vi "play_sysID_Z_Axis.vi"() -> ()   [LabVIEW 2017]
uses:
  sysID_Z-axis-params.ctl
  <vilib>/FPGAPlugInAG/cRIO-9082/niLvFpga_Open_cRIO-9082.vi
  <vilib>/rvi/interface/common/dynamic/niFpgaDynamicAddResources.vi
  <vilib>/FPGAPlugInAG/Dynamic/niLvFpga_Reset_Dynamic.vi
  <vilib>/rvi/interface/common/niFpgaWaitOnOcc.vi
  <vilib>/Utility/error.llb/Error Cluster From Error Code.vi
  <vilib>/rvi/errors/niLvFpgaAdjustHostInterfaceError.vi
  <vilib>/FPGAPlugInAG/Dynamic/niLvFpga_Run_Dynamic.vi
  <vilib>/FPGAPlugInAG/Dynamic/niLvFpga_Close_Dynamic.vi
  <vilib>/rvi/interface/nirviOpenFPGA/nirviOpenFPGA.xnode
  FPGA Bitfiles/afmimagingcontro_FPGATargetSPARTA_fpgasysIDZaxissi_jhd3Wt3fyx0.lvbitx
  <vilib>/rvi/interface/nirviMethod/nirviMethod.xnode
  <vilib>/rvi/interface/nirviReadWriteControl/nirviReadWriteControl.xnode
  <vilib>/rvi/interface/nirviCloseFPGA/nirviCloseFPGA.xnode
  <vilib>/FPGAPlugInAG/Dynamic/niLvFpga_ConfigureFifo_Dynamic.vi
  <vilib>/rvi/errors/niLvFpgaMergeErrorWithErrorCode.vi
  NiFpgaLv.dll
  <vilib>/rvi/interface/Simulation/niFpgaSimulationCallBeginRW.vi
panel:
  in  "Tab Control":enum32{"Main Control", "Debug Info"}(tab)
  in  "z-axis-settings":T1={"TOL"=0.3, "ramp-rate"=-5e-05, "z-u-max"=5.0, "offset"=0.0, "Ki"=0.001, "Z-error-threshold"=0.2, "Z-settled-samples\nthreshold "=200, "z_UP"=1.5, "zup-N"=5000} {"Z-error-threshold" format="%#_13g"; "ramp-rate" format="%#_4g"; "TOL" format="%#_13g"}
  in  "Z up":fxp<+/-,16,5>
  in  "trigger-0":bool
  in  "ABORT":bool
  out "Current Freq":dbl format="%#_13g"
  in  "Input Folder":path=path "C:/Users/arnold/Documents/MATLAB/AFM_SS/System_Identification/data/data_ZAxis"
  out "dataIn Path":path
  out "num_freqs":i32
  in  "input-file-name":string="z-axis_sines_in_299.csv"
  out "Input-meta-data-path":path
  out "output-data-path":path
  in  "overwrite":bool
  in  "note-blob":string
  out "Elements Remaining":i32=1
  out "Nsamps_i":i32
  out "size(s)":i32
  out "Current Case":i16
  out "log fifo num":i16
  out "input fifo num":i16
  out "error":errorcluster
  out "boolean  indicators 2":T2
  out "uzk)":dbl[](graph)
  out "z-err(k)":dbl[](graph)
  out "freqs":dbl[](array[numeric])
  out "ref(k) Signal":dbl[](graph)
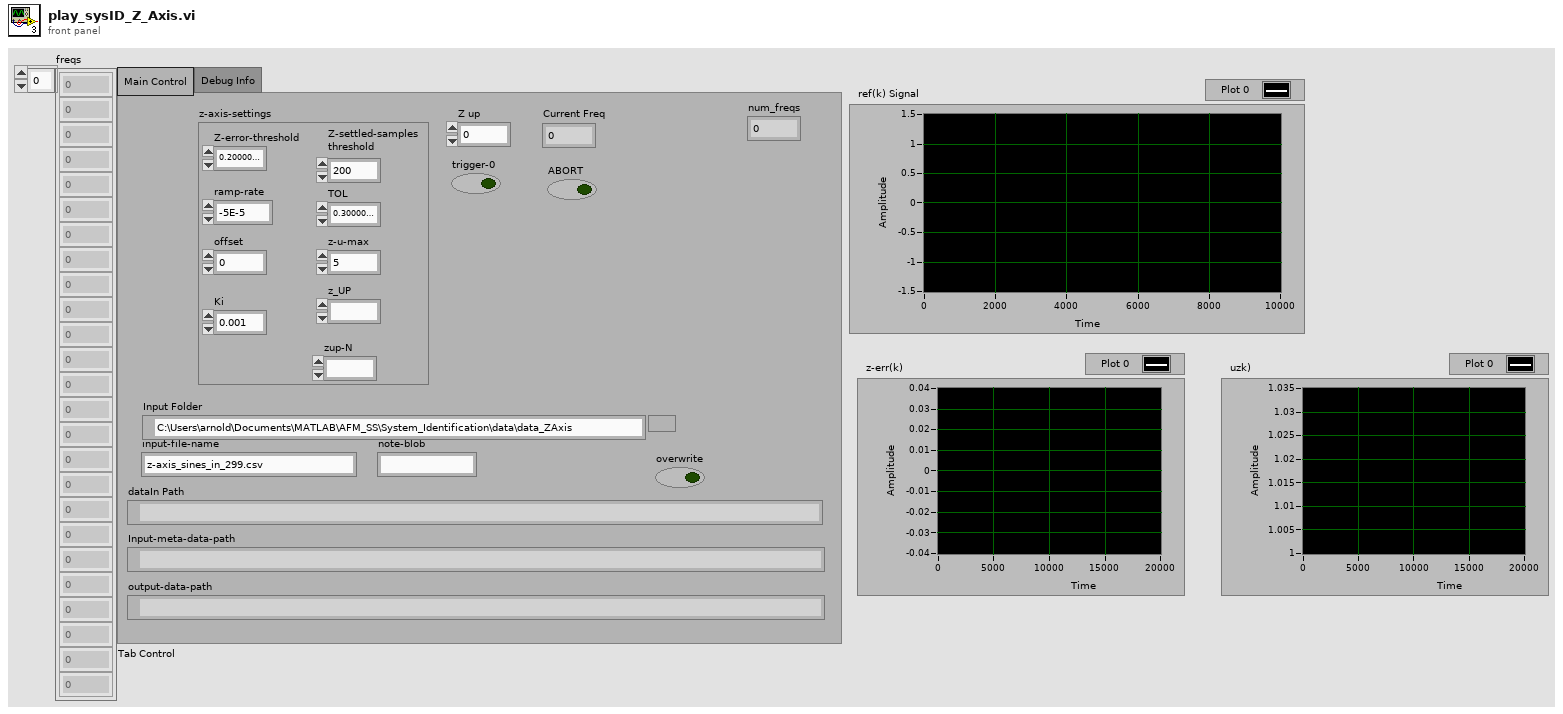
[diagram p1: front panel]
types:
  T1 = typedef "sysID_Z-axis-params.ctl" = cluster{"TOL":sgl, "ramp-rate":sgl, "z-u-max":sgl, "offset":sgl, "Ki":sgl, "Z-error-threshold":sgl, "Z-settled-samples\nthreshold ":i16, "z_UP":fxp<+/-,16,5>, "zup-N":i16}
  T2 = cluster{"unstable-z-traj":bool, "input fifo time-out":bool, "logging fifo timeout":bool, "scanning finished":bool, "unstable-x-traj":bool, "unstable-y-traj":bool, "ABORT":bool, "All Measurements Done":bool}
  T3 = typedef "sysID_ControlParams.ctl" = cluster{"Kp":sgl, "Umax ":sgl, "ymax":sgl, "TsTicks":u32, "z1":sgl, "num":sgl[], "den":sgl[], "TF Order":u8}
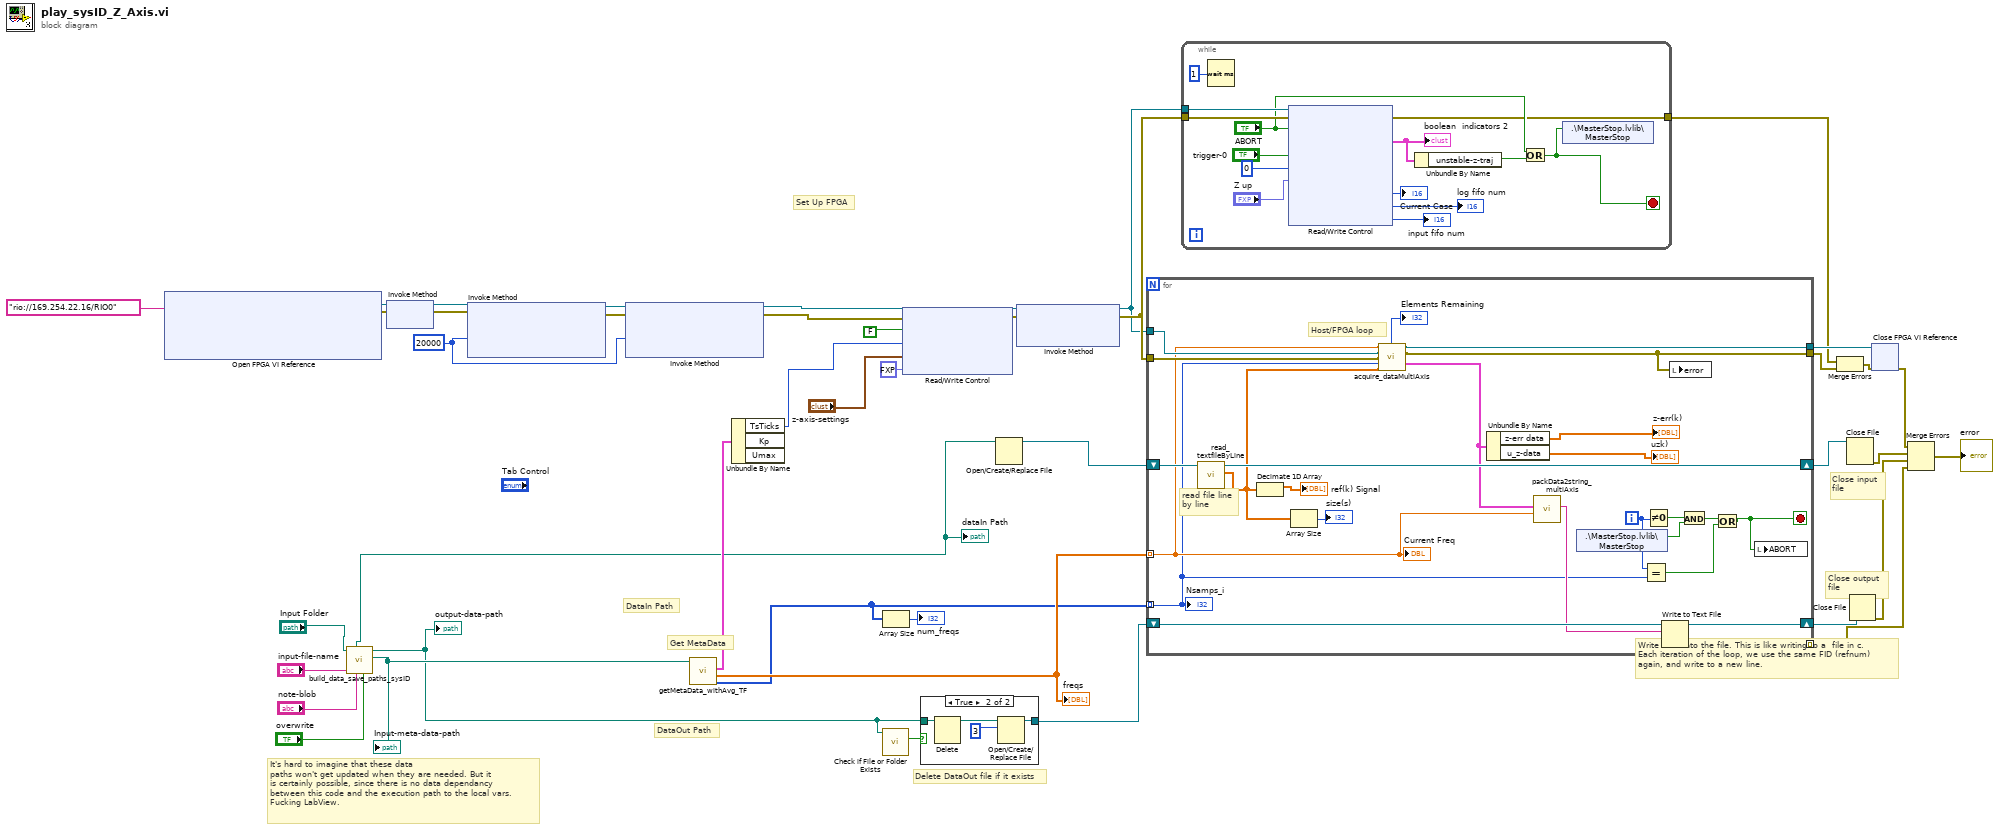
[diagram p0: block diagram]
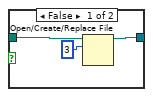
[diagram p2: hidden frame]
diagram:
  w14 = 20000 ("requested depth")
  # "It's hard to imagine that these data\npaths won't get updated when they are needed. But it \nis certainly possible, since there is no data dependancy \nbetween this code and the execution path to the local vars.\nFucking LabView."
  # "Set Up FPGA"
  # "Delete DataOut file if it exists"
  # "Close output\nfile"
  # "Close input\nfile"
  # "Write data into the file. This is like writing to a  file in c.\nEach iteration of the loop, we use the same FID (refnum) \nagain, and write to a new line."
  # "DataIn Path"
  # "DataOut Path"
  # "Get MetaData"
  n1 = xnode "Open FPGA VI Reference"("resource name"=tag "rio://169.254.22.16/RIO0") -> ("FPGA VI Reference Out"=w23:refnum<k20>, "error out"=w22:errorcluster)  [unwired: 1 in]
  n2 = call "build_data_save_paths_sysID.vi"("overwrite"="overwrite", "note-blob"="note-blob", "base-file-name"="input-file-name", "data-root"="Input Folder") -> ("output-meta-data-path"=w2:path, "output-data-path"=w1:path, "input-data-path"=w3:path)  [unwired: 4 in, 1 out]
  "dataIn Path" <- w3
  "Input-meta-data-path" <- w2
  "output-data-path" <- w1
  n3 = xnode "Invoke Method"("FPGA VI Reference In"=w23, "error in"=w22) -> ("FPGA VI Reference Out"=w27:refnum<k20>, "error out"=w26:errorcluster)
  n4 = xnode "Invoke Method"("FPGA VI Reference In"=w27, "error in"=w26, "Requested Depth"=w14) -> ("FPGA VI Reference Out"=w25:refnum<k20>, "error out"=w24:errorcluster)  [unwired: 1 out]
  n5 = xnode "Invoke Method"("FPGA VI Reference In"=w25, "error in"=w24, "Requested Depth"=w14) -> ("FPGA VI Reference Out"=w21:refnum<k20>, "error out"=w20:errorcluster)  [unwired: 1 out]
  n6 = call "getMetaData_withAvg_TF.vi"("MetaDataPath"=w2) -> ("Num Samples"=w9:i32[], "freqs (hz)"=w31:dbl[], "ControlParams"=w19:T3)  [unwired: 7 in]
  "freqs" <- w31
  n7 = Unbundle By Name(w19) -> ("TsTicks"=w15:u32)  [unwired: 2 out]
  n8 = call <vilib>:"Check if File or Folder Exists.vi"("path"=w1) -> ("file or folder exists?"=w28:bool)  [unwired: 8 in, 2 out]
  n9 = Array Size(array=w9) -> (size(s)=→"num_freqs":i32)
  n10 = xnode "Read/Write Control"("FPGA VI Reference In"=w21, "error in"=w20, "ABORT"=FALSE, "TsTicks"=w15, "sysID_Z_axis_params"="z-axis-settings", "init Z up"=fxp<+/-,16,5> 0.0) -> ("FPGA VI Reference Out"=w42:refnum<k20>, "error out"=w43:errorcluster)
  n11 = case shown="True" w28 {
    tunnel: w1 -> [w45 w50]
    tunnel: [w44 w48] -> w32
    frame False {
      n12 = Open/Create/Replace File(file path (use dialog)=w45, operation (0:open)=3) -> (refnum out=w44:refnum<file>)  [unwired: 4 in, 2 out]
    }
    frame True {
      n13 = Delete(path (use dialog)=w50) -> (deleted path=w49:path)  [unwired: 4 in, 2 out]
      n14 = Open/Create/Replace File(file path (use dialog)=w49, operation (0:open)=3) -> (refnum out=w48:refnum<file>)  [unwired: 4 in, 2 out]
    }
  }
  n15 = Open/Create/Replace File(file path (use dialog)=w3) -> (refnum out=w38:refnum<file>)  [unwired: 5 in, 2 out]
  n16 = xnode "Invoke Method"("FPGA VI Reference In"=w42, "error in"=w43) -> ("FPGA VI Reference Out"=w17:refnum<k20>, "error out"=w18:errorcluster)  [unwired: 1 in]
  n17 = for {
    tunnel: [w68] -> w41
    tunnel: [w58] -> w10
    tunnel: w18 -> [w66]
    tunnel: w17 -> [w67]
    tunnel: w31 -> [w64] mode=indexing
    shift-right: [w75] -> w40
    shift-left: w32 -> [w74]
    shift-right: [w73] -> w39
    shift-left: w38 -> [w72]
    tunnel: w9 -> [w52] mode=indexing
    tunnel: [w70] -> w33 mode=indexing
    i -> [w53]
    stop <- w54 stop-if-true
    # "Host/FPGA loop"
    # "read file line\nby line"
    n18 = call "read_textfileByLine.vi"("Byte Stream File in"=w72) -> ("Array"=w59:dbl[], "Byte Stream File out"=w73:refnum<file>)  [unwired: 9 in]
    n19 = Decimate 1D Array(w59) -> (→"ref(k) Signal":dbl[])  [unwired: 1 out]
    n20 = Array Size(array=w59) -> (size(s)=→"size(s)":i32)
    n21 = call "acquire_dataMultiAxis.vi"("Freq_i"=w64, "FPGA VI Reference in"=w67, "error in"=w66, "Nsamps_i"=w52, "data (sin wave) in"=w59) -> ("Elements Remaining"=→"Elements Remaining":i32, "FPGA VI Reference Out"=w68:refnum<k20>, "error IO"=w58:errorcluster, "output cluster"=w63:cluster{"z-err data":dbl[], "u_z-data":dbl[]})  [unwired: 6 in, 1 out]
    n22 = Unbundle By Name(w63) -> ("z-err data"=→"z-err(k)":dbl[], "u_z-data"=→"uzk)":dbl[])
    n23 = call "packData2string_multiAxis.vi"("F_i: current freq"=w64, "output cluster"=w63) -> ("spreadsheet string"=w65:string)  [unwired: 9 in]
    n24 = shared-variable ".\\MasterStop.lvlib\\MasterStop"() -> (w56:bool)  [unwired: 1 in, 1 out]
    n25 = Equal?(x=w53, y=w52) -> (x = y?=w51:bool)
    n26 = Not Equal To 0?(x=w53) -> (x != 0?=w57:bool)
    n27 = Write to Text File(file (use dialog)=w74, text=w65) -> (refnum out=w75:refnum<file>, error out=w70:errorcluster)  [unwired: 2 in, 1 out]
    n28 = local write "error"(w58) -> ()
    n29 = And(x=w57, y=w56) -> (x .and. y?=w55:bool)
    n30 = Or(x=w55, y=w51) -> (x .or. y?=w54:bool)
    n31 = local write "ABORT"(w54) -> ()
    "Current Freq" <- w64
    "Nsamps_i" <- w52
  }
  n32 = while {
    tunnel: w17 -> [w88]
    tunnel: w18 -> [w87]
    tunnel: [w77] -> w11
    stop <- w76 stop-if-true
    n33 = Wait (ms)(milliseconds to wait=u32 1) -> ()  [unwired: 1 out]
    n34 = xnode "Read/Write Control"("FPGA VI Reference In"=w88, "error in"=w87, "ABORT"="ABORT", "trigger-0"="trigger-0", "initial case"=i16 0, "init Z up"="Z up") -> ("error out"=w77:errorcluster, "boolean  indicators"=w83:T2, "Current Case"=→"Current Case":i16, "Numeric"=→"log fifo num":u32, "Numeric 2"=→"input fifo num":u32)  [unwired: 1 out]
    "boolean  indicators 2" <- w83
    n35 = Unbundle By Name(w83) -> ("unstable-z-traj"=w82:bool)
    n36 = Or(x="ABORT", y=w82) -> (x .or. y?=w76:bool)
    n37 = shared-variable ".\\MasterStop.lvlib\\MasterStop"(w76) -> ()  [unwired: 1 in, 1 out]
  }
  n38 = Merge Errors(w11, w10) -> (w12:errorcluster)
  n39 = Close File(refnum=w39) -> (error out=w36:errorcluster)  [unwired: 1 in, 1 out]
  n40 = Close File(refnum=w40) -> (error out=w37:errorcluster)  [unwired: 1 in, 1 out]
  n41 = xnode "Close FPGA VI Reference"("FPGA VI Reference In"=w41, "error in"=w12) -> ("error out"=w34:errorcluster)
  n42 = Merge Errors(w34, w36, w37, w33) -> (→"error":errorcluster)
